vi "From Serial Form.vi"(6 "Serial Version":T1, 10 "Deserializer in":refnum<class "Deserializer.lvclass">, 11 "cPAS in":refnum<class "cPAS.lvclass">) -> (0 "error out":errorcluster, 2 "Deserializer out":refnum<class "Deserializer.lvclass">, 3 "cPAS out":refnum<class "cPAS.lvclass">)   [LabVIEW 2012]
uses:
  Reusable/PAS/Data/Main/PAS Data.lvclass
  Data/cPAS Data.lvclass
  Data/cPAS Cell Data/cPAS Cell Data.lvclass
  <userlib>/Serialization/Serializable/Serializable.lvclass
  Reusable/Serial IO/Serial IO.lvclass
  <userlib>/Serialization/Serializable/Remove Serializable.vi
  <userlib>/Serialization/Serializable/Remove Single Array.vi
  <userlib>/Serialization/Serializable/Remove Single.vi
  <userlib>/Serialization/Serializable/Remove Boolean.vi
  <userlib>/Serialization/Serializable/Remove Boolean Array.vi
  cPAS.lvclass
  Reusable/PAS/Data/Cell/PAS Cell Data.lvclass
  <userlib>/Serialization/Serialization Common/Serial Version.ctl
  <userlib>/Serialization/Serialization Common/Serialization Common.lvlib
  <userlib>/Serialization/Deserializer/Deserializer.lvclass
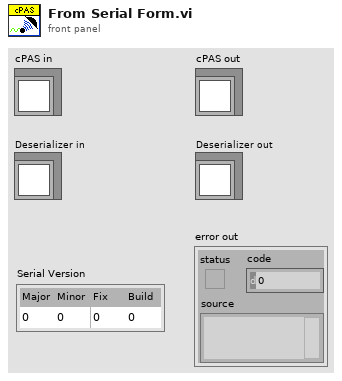
[diagram p1: front panel]
types:
  T1 = typedef "Serialization Common.lvlib/Serial Version.ctl" = cluster{"Major":u16, "Minor":u16, "Fix":u16, "Build":u16}
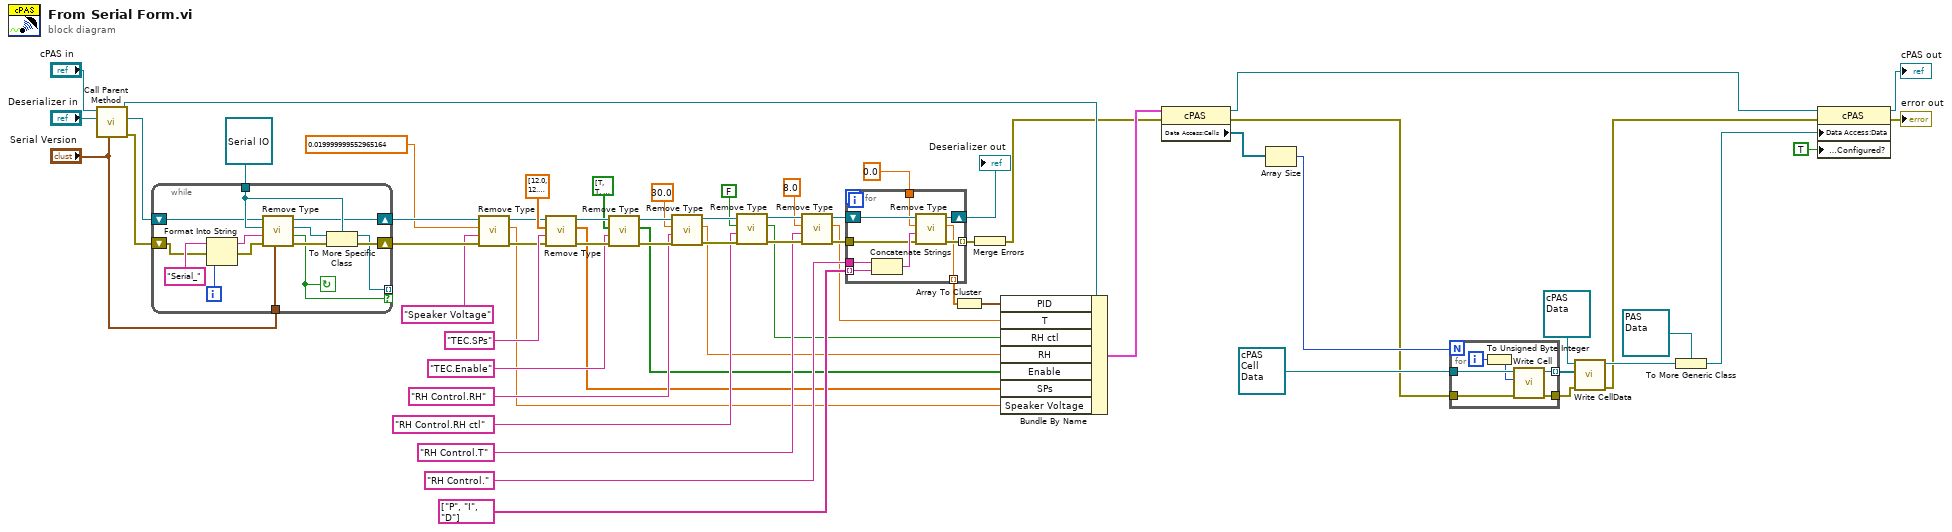
[diagram p0: block diagram]
diagram:
  n1 = call-parent "Call Parent Method"("Serial Version"="Serial Version", "Deserializer in"="Deserializer in", "PAS in"="cPAS in") -> ("error out"=w55:errorcluster, "Deserializer out"=w59:refnum<class "Deserializer.lvclass">, "PAS out"=w27:refnum<class "cPAS.lvclass">)  [unwired: 6 in]
  n2 = while {
    shift-right: [w74] -> w18
    shift-left: w55 -> [w67]
    shift-right: [w70] -> w19
    shift-left: w59 -> [w72]
    tunnel: refnum<class "Serial IO.lvclass"> refnum ("Serial IO.lvclass") -> [w73]
    tunnel: [w71] -> _ mode=indexing if=w64
    tunnel: "Serial Version" -> [w65]
    i -> [w77]
    stop <- w64 continue-if-true
    n3 = Format Into String(initial string="Serial_", error in=w67, w77) -> (resulting string=w76:string, error out=w66:errorcluster)  [unwired: 1 in]
    n4 = call-poly <userlib>:"Remove Type.vi"("Serial Version"=w65, "error in (no error)"=w66, "Name"=w76, "Default Value"=w73, "Deserializer in"=w72) -> ("error out"=w75:errorcluster, "Found?"=w64:bool, "Serializable"=w69:refnum<class "Serializable.lvclass">, "Deserializer out"=w70:refnum<class "Deserializer.lvclass">)  [unwired: 3 in]
    n5 = To More Specific Class(target class=w73, reference=w69, error in=w75) -> (specific class reference=w71:refnum<class "Serial IO.lvclass">, error out=w74:errorcluster)
  }
  n6 = call-poly <userlib>:"Remove Type.vi"("error in (no error)"=w18, "Name"="Speaker Voltage", "Default Value"=sgl 0.02, "Deserializer in"=w19) -> ("error out"=w17:errorcluster, "Numeric"=w13:sgl, "Deserializer out"=w16:refnum<class "Deserializer.lvclass">)  [unwired: 4 in, 1 out]
  n7 = call-poly <userlib>:"Remove Type.vi"("error in (no error)"=w17, "Name"="TEC.SPs", "Default Value"=sgl[] [12.0, 12.0, 12.0, 12.0, 12.0], "Deserializer in"=w16) -> ("error out"=w47:errorcluster, "Singles"=w12:sgl[], "Deserializer out"=w48:refnum<class "Deserializer.lvclass">)  [unwired: 4 in, 1 out]
  n8 = call-poly <userlib>:"Remove Type.vi"("error in (no error)"=w47, "Name"="TEC.Enable", "Default Value"=bool[] [TRUE, TRUE, TRUE, TRUE, TRUE], "Deserializer in"=w48) -> ("error out"=w43:errorcluster, "Booleans"=w11:bool[], "Deserializer out"=w44:refnum<class "Deserializer.lvclass">)  [unwired: 4 in, 1 out]
  n9 = call-poly <userlib>:"Remove Type.vi"("error in (no error)"=w43, "Name"="RH Control.RH", "Default Value"=sgl 30.0, "Deserializer in"=w44) -> ("error out"=w39:errorcluster, "Numeric"=w23:sgl, "Deserializer out"=w40:refnum<class "Deserializer.lvclass">)  [unwired: 4 in, 1 out]
  n10 = call-poly <userlib>:"Remove Type.vi"("error in (no error)"=w39, "Name"="RH Control.RH ctl", "Default Value"=FALSE, "Deserializer in"=w40) -> ("error out"=w35:errorcluster, "Boolean"=w24:bool, "Deserializer out"=w36:refnum<class "Deserializer.lvclass">)  [unwired: 4 in, 1 out]
  n11 = call-poly <userlib>:"Remove Type.vi"("error in (no error)"=w35, "Name"="RH Control.T", "Default Value"=sgl 8.0, "Deserializer in"=w36) -> ("error out"=w30:errorcluster, "Numeric"=w25:sgl, "Deserializer out"=w32:refnum<class "Deserializer.lvclass">)  [unwired: 4 in, 1 out]
  n12 = for {
    tunnel: w30 -> [w82]
    shift-right: [w81] -> w31
    shift-left: w32 -> [w83]
    tunnel: string[] ["P", "I", "D"] -> [w86] mode=indexing
    tunnel: "RH Control." -> [w85]
    tunnel: [w80] -> w51 mode=indexing
    tunnel: sgl 0.0 ("Default Value") -> [w79]
    tunnel: [w78] -> w28 mode=indexing
    n13 = Concatenate Strings(w85, w86) -> (w84:string)
    n14 = call-poly <userlib>:"Remove Type.vi"("error in (no error)"=w82, "Name"=w84, "Default Value"=w79, "Deserializer in"=w83) -> ("error out"=w80:errorcluster, "Numeric"=w78:sgl, "Deserializer out"=w81:refnum<class "Deserializer.lvclass">)  [unwired: 4 in, 1 out]
  }
  "Deserializer out" <- w31
  n15 = Array To Cluster(array=w28) -> (cluster=w26:cluster{"[0]":sgl, "[1]":sgl, "[2]":sgl})
  n16 = Merge Errors(w51) -> (w21:errorcluster)
  n17 = Bundle By Name(cluster=w27, "PID"=w26, "T"=w25, "RH ctl"=w24, "RH"=w23, "Enable"=w11, "SPs"=w12, "Speaker Voltage"=w13) -> (w22:cluster{})
  n18 = property class="cPAS"(reference=w22, error in=w21) -> (reference out=w57:refnum<class "cPAS.lvclass">, error out=w2:errorcluster, "Data Access:Cells"=w61:refnum<class "PAS Cell.lvclass">[])
  n19 = Array Size(array=w61) -> (size(s)=w4:i32)
  n20 = for {
    N: w4 -> [_]
    tunnel: refnum<class "cPAS Cell Data.lvclass"> refnum ("cPAS Cell") -> [w92]
    tunnel: [w91] -> w10 mode=indexing
    tunnel: [w88] -> w9
    tunnel: w2 -> [w87]
    i -> [w90]
    n21 = To Unsigned Byte Integer(number=w90) -> (unsigned 8bit integer=w89:u8)
    n22 = call "Write Cell.vi"("error in"=w87, "Cell"=w89, "PAS Cell Data in"=w92) -> ("error out"=w88:errorcluster, "PAS Cell Data out"=w91:refnum<class "cPAS Cell Data.lvclass">)  [unwired: 7 in]
  }
  n23 = call "Write CellData.vi"("error in"=w9, "CellData"=w10, "PAS Data in"=refnum<class "cPAS Data.lvclass"> refnum ("cPAS Data")) -> ("error out"=w1:errorcluster, "PAS Data out"=w6:refnum<class "cPAS Data.lvclass">)  [unwired: 7 in]
  n24 = To More Generic Class(target class=refnum<class "PAS Data.lvclass"> refnum ("Data"), reference=w6) -> (generic class reference=w3:refnum<class "PAS Data.lvclass">)
  n25 = property class="cPAS"(reference=w57, error in=w1, "Data Access:Data"=w3, "Data Access:Configured?"=TRUE ("Configured?")) -> (reference out=→"cPAS out":refnum<class "cPAS.lvclass">, error out=→"error out":errorcluster)
